vi "build_query_insert.vi"(4 "Problem":string, 6 "Item Description":string, 7 "Call No.":string, 9 "Customer Contact No.":string, 10 "Customer":string, 11 "Engineer Name":string) -> (3 "result string":string)   [LabVIEW 2023]
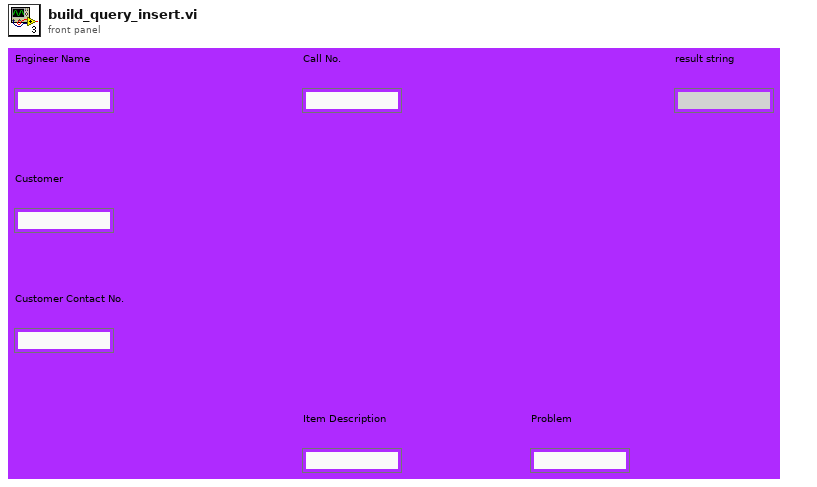
[diagram p1: front panel]
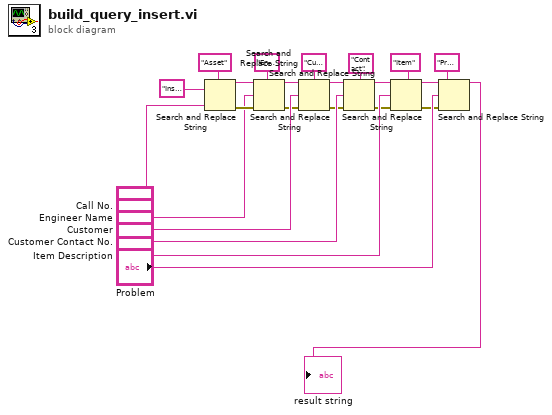
[diagram p0: block diagram]
diagram:
  n1 = Search and Replace String(input string="Insert into Service_Calls_Entry values\n('Asset', GETDATE(), 'Engineer', 'Customer', 'Contact', 'Item', 'Problem','Pending')", search string="Asset", replace string="Call No.") -> (result string=w5:string, error out=w14:errorcluster)  [unwired: 5 in, 2 out]
  n2 = Search and Replace String(input string=w5, search string="Engineer", replace string="Engineer Name", error in=w14) -> (result string=w6:string, error out=w15:errorcluster)  [unwired: 4 in, 2 out]
  n3 = Search and Replace String(input string=w6, search string="Customer", replace string="Customer", error in=w15) -> (result string=w7:string, error out=w2:errorcluster)  [unwired: 4 in, 2 out]
  n4 = Search and Replace String(input string=w7, search string="Contact", replace string="Customer Contact No.", error in=w2) -> (result string=w8:string, error out=w3:errorcluster)  [unwired: 4 in, 2 out]
  n5 = Search and Replace String(input string=w8, search string="Item", replace string="Item Description", error in=w3) -> (result string=w9:string, error out=w4:errorcluster)  [unwired: 4 in, 2 out]
  n6 = Search and Replace String(input string=w9, search string="Problem", replace string="Problem", error in=w4) -> (result string=→"result string":string)  [unwired: 4 in, 3 out]
